vi "Close.vi"(11 "FpgaRef5782 In":refnum<class "FpgaRefx410.lvclass">) -> ()   [LabVIEW 2025, in "FpgaRefx410.lvclass"]
uses:
  FpgaRefx410.lvclass
  FpgaRefx410.lvclass/FpgaRefx410.ctl
  <vilib>/FPGAPlugInAG/Dynamic/niLvFpga_Close_Dynamic.vi
  FpgaRefBase/FpgaRefBase.lvclass
  <vilib>/rvi/interface/nirviCloseFPGA/nirviCloseFPGA.xnode
  x410 FPGA ref.ctl
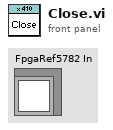
[diagram p1: front panel]
types:
  T1 = typedef "x410 FPGA ref.ctl" = refnum<k20>
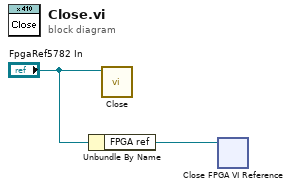
[diagram p0: block diagram]
diagram:
  n1 = Unbundle By Name("FpgaRef5782 In") -> ("FPGA ref"=w1:T1)
  n2 = call-parent "Close.vi"("FpgaRefBase In"="FpgaRef5782 In") -> ()  [unwired: 11 in]
  n3 = xnode "Close FPGA VI Reference"("FPGA VI Reference In"=w1) -> ()  [unwired: 1 in, 1 out]
